vi "Command Type.vi"(11 "Save Var Command Config in":refnum<class "Save Var Command Config.lvclass">) -> (2 "Command Type":T1)   [LabVIEW 2020, in "VolatusSeqConfig.lvlib" / "Save Var Command Config.lvclass"]
uses:
  Save Var Command Config.lvclass
  Save Var Command Config.lvclass/Save Var Command Config.ctl
  Command Type.ctl
  VolatusSeqConfig.lvlib
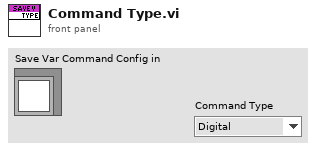
[diagram p1: front panel]
types:
  T1 = typedef "VolatusSeqConfig.lvlib/Command Type.ctl" = enum16{"Digital", "Numeric", "Transition", "Stop", "StartLog", "StopLog", "Start", "Event", "Error", "HTTP", "ResetVar", "IncVar", "DecVar", "SaveVar", "LoadVar", "AddVar", "SubVar"}
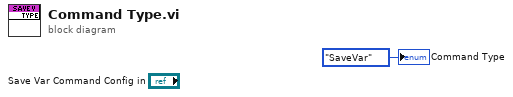
[diagram p0: block diagram]
diagram:
  "Command Type" <- Command_Type."SaveVar" ("Command Type")
